vi "DiffDriveTrainSim_Pack_Model_Params.vi"(4 "WheelRadius_M":dbl, 6 "TracWidth_M":dbl, 7 "DCMOTOR_TYPES":T1, 8 "Gearing":dbl, 9 "MOI kgm2":dbl, 10 "Mass kg":dbl, 11 "Num Motors":i32) -> (3 "DiffDriveSim_Model _Params":T2 {"MOI kgm2" format="%#_13g"; "Mass kg" format="%#_13g"; "Gearing" format="%#_13g"; "WheelRadius_M" format="%#_13g"; "TracWidth_M" format="%#_13g"})   [LabVIEW 2019, in "Trajectory_Library.lvlib"]
uses:
  Trajectory_Library.lvlib
  TypeDef/DIFF_DRIVE_SIM_MODEL_PARAMS.CTL
  Enum/DCMOTOR_TYPES_ENUM.ctl
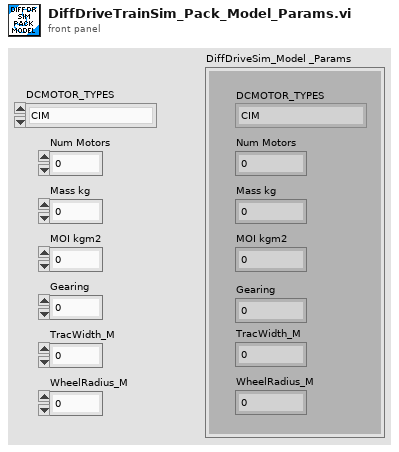
[diagram p1: front panel]
types:
  T1 = typedef "Trajectory_Library.lvlib/DCMOTOR_TYPES_ENUM.ctl" = enum16{"CIM", "AndyMark 9015", "Andy Mark RS 775 125", "Bag", "BaneBots RS 550", "BaneBots RS 775", "Falcon 500", "Mini CIM", "NEO", "NEO 550", "Romi BuiltIn", "Vex 775 Pro", "Snow Blower AM 2235A", "Bosch Seat AM 3493"}
  T2 = typedef "Trajectory_Library.lvlib/DIFF_DRIVE_SIM_MODEL_PARAMS.CTL" = cluster{"TracWidth_M":dbl, "WheelRadius_M":dbl, "Gearing":dbl, "Mass kg":dbl, "MOI kgm2":dbl, "DCMOTOR_TYPES":T1, "Num Motors":i32}
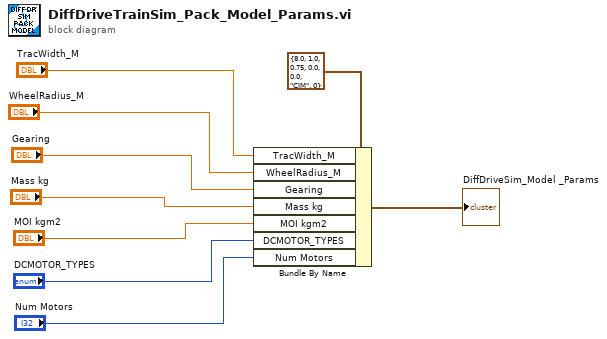
[diagram p0: block diagram]
diagram:
  n1 = Bundle By Name(cluster=T2 {"TracWidth_M"=8.0, "WheelRadius_M"=1.0, "Gearing"=0.75, "Mass kg"=0.0, "MOI kgm2"=0.0, "DCMOTOR_TYPES"=enum."CIM", "Num Motors"=0} ("SngJntArmSim_Simulation _Params"), "TracWidth_M"="TracWidth_M", "WheelRadius_M"="WheelRadius_M", "Gearing"="Gearing", "Mass kg"="Mass kg", "MOI kgm2"="MOI kgm2", "DCMOTOR_TYPES"="DCMOTOR_TYPES", "Num Motors"="Num Motors") -> (→"DiffDriveSim_Model _Params":T2)
